vi "HSVCycle.vi"(10 "milliseconds to wait":u32=25, 11 "Hue":dbl) -> (3 "Hue Out":dbl)   [LabVIEW 2017]
uses:
  <vilib>/myRIO/Express VI/Onboard IO/PWM/PWM Express VI.xnode
  <vilib>/myRIO/Instrument Drivers/Onboard IO/PWM/typedefs/PWM Reference.ctl
  <vilib>/myRIO/Instrument Drivers/Onboard IO/PWM/PWM.lvlib
  <vilib>/myRIO/Instrument Drivers/Onboard IO/PWM/typedefs/PWM Configuration.ctl
  <vilib>/myRIO/Common/Instrument Driver Framework/myRIO v1.0/PWM/typedefs/PWM Channels Enum.ctl
  <vilib>/myRIO/Common/Instrument Driver Framework/Utilities/typedefs/myRIO Generic Hardware Reference.ctl
  <vilib>/myRIO/Common/Instrument Driver Framework/Utilities/typedefs/myRIO v1.0 Reference.ctl
  <vilib>/myRIO/Common/Instrument Driver Framework/Utilities/typedefs/Generic FPGA Reference.ctl
  <vilib>/myRIO/Common/Instrument Driver Framework/Utilities/typedefs/Hardware Version Enum.ctl
  <vilib>/myRIO/Instrument Drivers/Onboard IO/PWM/vis/Set Duty Cycle and Frequency.vi
  <vilib>/myRIO/Instrument Drivers/Onboard IO/PWM/vis/myRIO PWM Open.xnode
  <vilib>/userdefined/High Color/nirio_resource_hc.ctl
  <vilib>/myRIO/Common/Instrument Driver Framework/myRIO v1.0/PWM/vis/myRIO v1.1 Open PWM.vi
  <vilib>/myRIO/Common/Instrument Driver Framework/Utilities/vis/Is FPGA Ref Available.vi
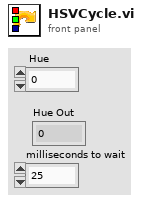
[diagram p1: front panel]
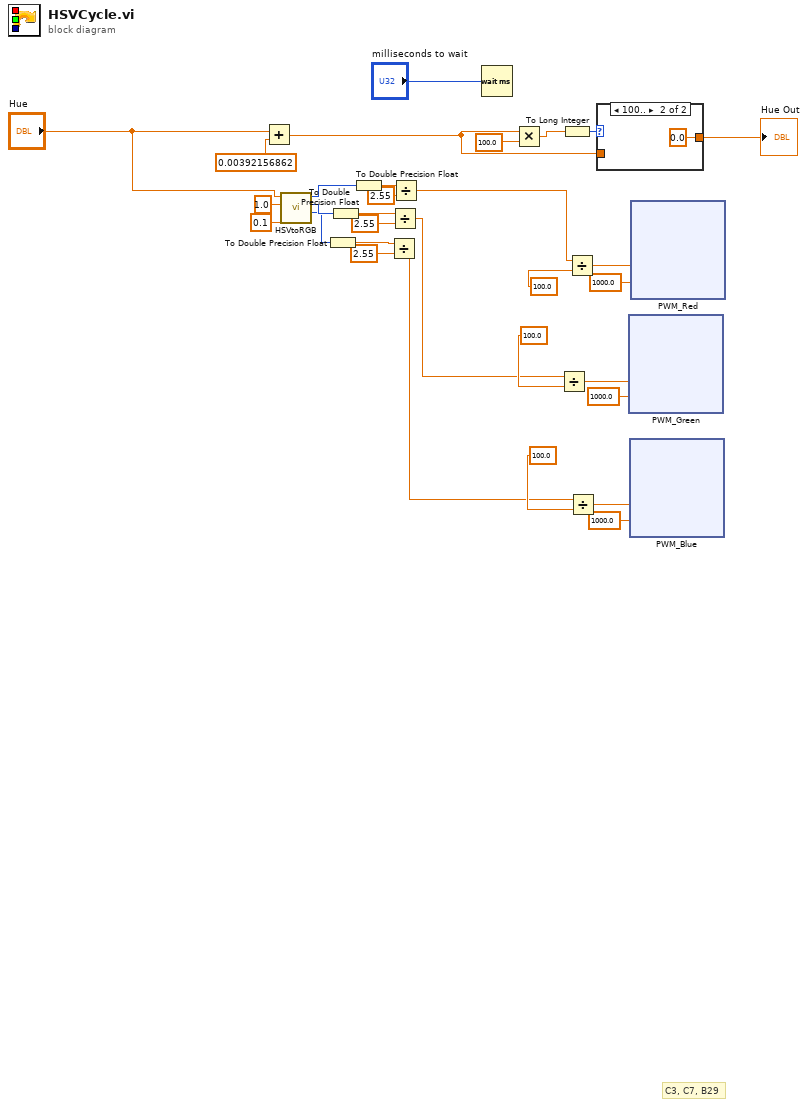
[diagram p0: block diagram]
diagram:
  # "C3, C7, B29"
  n1 = Add(x="Hue", y=0.00392156862) -> (x+y=w19:dbl)
  n2 = call "HSVtoRGB.vi"("Value"=0.1, "Saturation"=1.0, "Hue [0-1)"="Hue") -> ("Blue"=w29:u8, "Green"=w30:u8, "Red"=w31:u8)  [unwired: 6 in]
  n3 = To Double Precision Float(number=w29) -> (double precision float=w26:dbl)
  n4 = To Double Precision Float(number=w30) -> (double precision float=w27:dbl)
  n5 = To Double Precision Float(number=w31) -> (double precision float=w28:dbl)
  n6 = Divide(x=w26, y=2.55) -> (x/y=w4:dbl)
  n7 = Divide(x=w27, y=2.55) -> (x/y=w5:dbl)
  n8 = Divide(x=w28, y=2.55) -> (x/y=w6:dbl)
  n9 = Wait (ms)(milliseconds to wait="milliseconds to wait") -> ()  [unwired: 1 out]
  n10 = Multiply(x=w19, y=100.0 ("x")) -> (x*y=w17:dbl)
  n11 = Divide(x=w5, y=100.0) -> (x/y=w14:dbl)
  n12 = To Long Integer(number=w17) -> (32bit integer=w16:i32)
  n13 = Divide(x=w6, y=100.0) -> (x/y=w13:dbl)
  n14 = Divide(x=w4, y=100.0) -> (x/y=w15:dbl)
  n15 = case shown="100.." w16 {
    tunnel: w19 -> [w32 _]
    tunnel: [w32 0.0] -> w3
    frame 0, Default {
    }
    frame 100.. {
    }
  }
  "Hue Out" <- w3
  n16 = xnode "PWM_Green"("Duty Cycle"=w14, "Frequency [Hz]"=1000.0) -> ()  [unwired: 1 in, 1 out]
  n17 = xnode "PWM_Blue"("Duty Cycle"=w15, "Frequency [Hz]"=1000.0) -> ()  [unwired: 1 in, 1 out]
  n18 = xnode "PWM_Red"("Duty Cycle"=w13, "Frequency [Hz]"=1000.0) -> ()  [unwired: 1 in, 1 out]
